vi "L0_Sum_Adder.vi"() -> ()   [LabVIEW 2009]
uses:
  Program Files/National Instruments/LabVIEW 2012/instr.lib/Agilent 8000 Series/Public/Configure/Configure Math (Binary Operation).vi
  <vilib>/Utility/file.llb/Write To Spreadsheet File (string).vi
  Program Files/National Instruments/LabVIEW 2012/instr.lib/Agilent 8000 Series/Public/Data/Low Level/Fetch Measurement (More).vi
  Program Files/National Instruments/LabVIEW 2012/instr.lib/Agilent 8000 Series/Agilent 8000 Series.lvlib
panel:
  in  "Channels Combinations":i32[](array[numeric])=[3, 12, 48, 96, 7, 28, 112, 15, 120, 31, 124, 63, 126, 127]
  out "error out":errorcluster={"status"=TRUE, "code"=-1073807343, "source"="VISA Open in Agilent 81150.lvlib:Initialize.vi->Set_Gen_Conf.vi->L0_Sum_Adder.vi"}
  in  "Voltage Array":dbl[](array[numeric])=[0.2, 0.4, 0.6, 0.8]
  in  "Osc":refnum<visa-resource-name>="Oscilloscope"
  in  "Generator":refnum<visa-resource-name>="generadorpulsos"
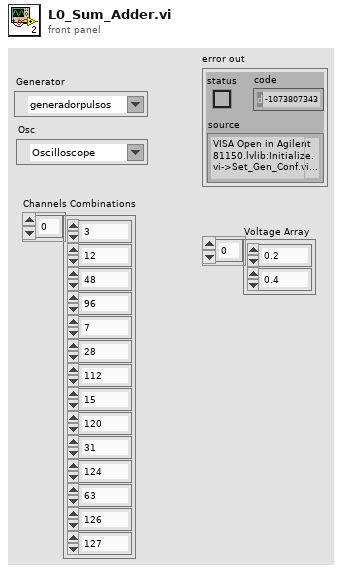
[diagram p1: front panel]
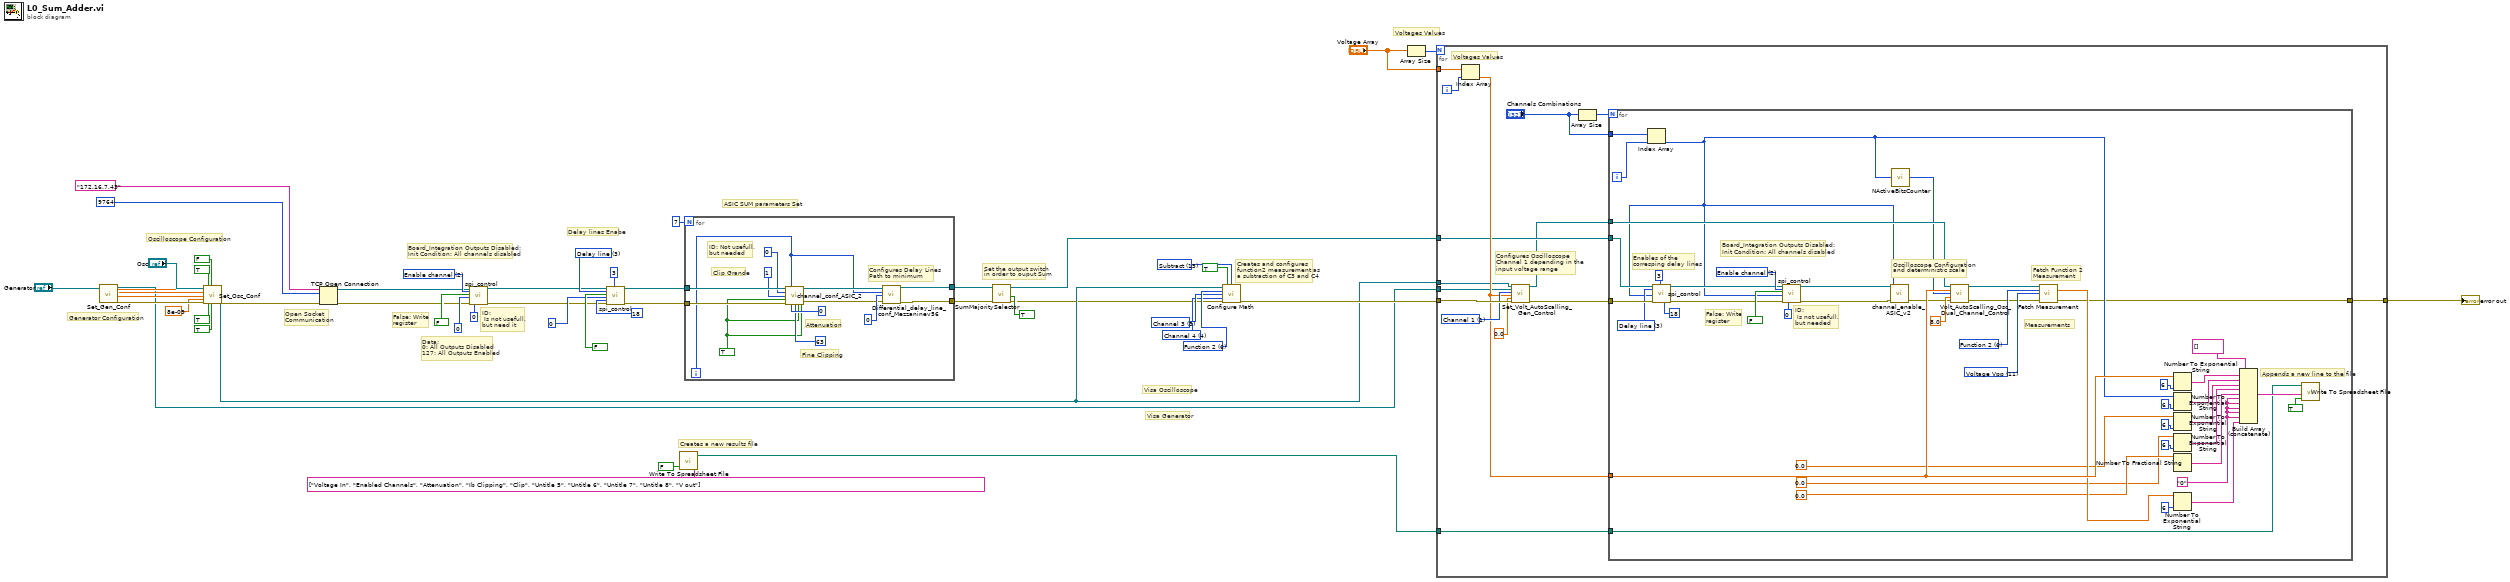
[diagram p0: block diagram]
diagram:
  w18 = u16 2 items=["Attenuation", "Clipping", "Enable channel", "Delay line", "ASIC"] ("Device")
  w21 = u16 3 items=["Attenuation", "Clipping", "Enable channel", "Delay line", "ASIC"] ("Device")
  w33 = u16 6 items=["Function 1"=5, "Function 2"=6, "Function 3"=7, "Function 4"=8] ("Math Channel (5: Function 1)")
  w34 = u16 15 items=["Add"=12, "Divide"=13, "Multiply"=14, "Subtract"=15, "Common Mode"=16, "Versus"=17] ("Math Operation (12: Add)")
  w32 = 3 items=["Channel 1"=1, "Channel 2"=2, "Channel 3"=3, "Channel 4"=4] ("Channel (1: Channel 1)")
  w31 = 4 items=["Channel 1"=1, "Channel 2"=2, "Channel 3"=3, "Channel 4"=4] ("Channel (1: Channel 1)")
  # "Creates and configures\nfunction2 measurement as\na subtraction of C3 and C4"
  # "Creates a new results file"
  # "Set the output switch\nin order to ouput Sum"
  # "ASIC SUM parameters Set"
  # "False: Write\nregister"
  # "Data:\n0: All Outputs Disabled\n127: All Outputs Enabled"
  # "ID:\n Is not usefull, \nbut need it"
  # "Board_Integration Outputs Disabled:\nInit Condition: All channels disabled"
  # "Delay lines Enabe"
  # "Open Socket\nCommunication"
  # "Visa Generator"
  # "Visa Oscilloscope"
  # "Oscilloscope Configuration"
  # "Voltages Values"
  # "Generator Configuration"
  n1 = call "Set_Gen_Conf.vi"("AWG VISA"="Generator") -> ("Amplitude 1 OUT"=w41:dbl, "VISA resource name out"=w26:refnum<visa-resource-name>, "Pulse Width in seconds 1 OUT"=w40:dbl, "Trigger Level 1"=w39:dbl, "error out"=w38:errorcluster)  [unwired: 11 in, 3 out]
  n2 = call "Set_Osc_Conf.vi"("VISA resource name"="Osc", "Amplitude IN"=w41, "Trigger Level IN"=w39, "Pulse Width in seconds IN"=w40, "Position 1"=8e-09, "error in (no error)"=w38, "Channel 1"=TRUE, "Channel 3"=TRUE, "Channel 2"=FALSE, "Channel 4"=TRUE) -> ("VISA resource name out"=w25:refnum<visa-resource-name>, "error out"=w15:errorcluster)  [unwired: 8 in]
  n3 = TCP Open Connection(address="172.16.7.43", remote port or service name=u16 9764, error in (no error)=w15) -> (connection ID=w14:refnum<k5>, error out=w13:errorcluster)  [unwired: 2 in]
  n4 = call "spi_control.vi"("connection ID"=w14, "Device"=w18, "Read/#write"=FALSE, "Data"=0, "error out 3"=w13, "Id in"=0) -> ("connection ID out"=w2:refnum<k5>, "error out 2"=w1:errorcluster)  [unwired: 6 in, 6 out]
  n5 = call "spi_control.vi"("connection ID"=w2, "Device"=w21, "Read/#write"=FALSE, "Data"=0, "Register or channel"=18, "error out 3"=w1, "chip delay"=3) -> ("connection ID out"=w11:refnum<k5>, "error out 2"=w12:errorcluster)  [unwired: 5 in, 6 out]
  n6 = call-poly <vilib>:"Write To Spreadsheet File.vi"("append to file? (new file:F)"=FALSE, "1D data"=string[] ["Voltage In", "Enabled Channels", "Attenuation", "Ib Clipping", "Clip", "Untitle 5", "Untitle 6", "Untitle 7", "Untitle 8", "V out"]) -> ("new file path (Not A Path if cancelled)"=w27:path)  [unwired: 6 in]
  n7 = for {
    N: 7 -> [_]
    tunnel: w12 -> [w62]
    tunnel: w11 -> [w61]
    tunnel: [w51] -> w7
    tunnel: [w52] -> w9
    i -> [w50]
    w56 = TRUE ("maj/sum")
    # "Configures Delay Lines\nPath to minimum"
    # "Attenuation"
    # "Fine Clipping"
    # "Clip Grande"
    # "ID: Not usefull,\nbut needed"
    n8 = call "channel_conf_ASIC_2.vi"("connection ID"=w61, "Ring"=w50, "Id in"=u32 0, "Clip_sel_b"=u32 1, "CompBuf_en_b"=w56, "error out"=w62, "Att gain"=u32 0, "Ib_ClipVb"=u32 63, "Clip_en_b"=w56, "Att_en_b"=w56) -> ("connection ID out"=w54:refnum<k5>, "error out 2"=w53:errorcluster)  [unwired: 1 in, 3 out]
    n9 = call "Differential_delay_line_conf_Mezzaninev56.vi"("connection ID"=w54, "channel"=w50, "Delay value"=u16 0, "error in (no error)"=w53) -> ("connection ID out"=w51:refnum<k5>, "error out 2"=w52:errorcluster)  [unwired: 4 in, 6 out]
  }
  n10 = call "SumMajoritySelector.vi"("On Sum\nOff Majority"=TRUE ("On Sum\nOff Majority"), "error in (no error)"=w9, "connection ID"=w7) -> ("error out"=w5:errorcluster, "connection ID out"=w6:refnum<k5>)  [unwired: 5 in]
  n11 = call-poly "Configure Math.vi"("VISA resource name"=w25, "Enable Math Channel (T:Enable)"=TRUE, "Math Operation (12: Add)"=w34, "Math Channel (5: Function 1)"=w33, "Math Operand (1: Channel 1)"=w32, "Math Operand (2: Channel 2)"=w31, "error in (no error)"=w5) -> ("error out"=w30:errorcluster)  [unwired: 7 in, 1 out]
  n12 = Array Size(array="Voltage Array") -> (size(s)=w37:i32)
  n13 = for {
    N: w37 -> [_]
    tunnel: w6 -> [w68]
    tunnel: w30 -> [w75]
    tunnel: "Voltage Array" -> [w77]
    tunnel: w27 -> [w72]
    tunnel: w26 -> [w70]
    tunnel: w25 -> [w69]
    tunnel: [w63] -> w3
    i -> [w76]
    w74 = 1 items=["Channel 1"=1, "Channel 2"=2, "Channel 3"=3, "Channel 4"=4] ("Channel")
    # "Configures Oscilloscope\nChannel 1 depending in the \ninput voltage range"
    # "Voltages Values"
    n14 = Index Array(array=w77, index=w76) -> (element=w73:dbl)
    n15 = call "Set_Volt_AutoScalling_Gen_Control.vi"("VISA Oscilloscope"=w69, "VISA Generator"=w70, "Channel"=w74, "Amplitude"=w73, "DC Offset"=0.0, "error in (no error)"=w75) -> ("VISA Oscilloscope"=w66:refnum<visa-resource-name>, "error out"=w67:errorcluster)  [unwired: 11 in, 1 out]
    n16 = Array Size(array="Channels Combinations") -> (size(s)=w65:i32)
    n17 = for {
      N: w65 -> [_]
      tunnel: w68 -> [w96]
      tunnel: w73 -> [w104]
      tunnel: w72 -> [w105]
      tunnel: w67 -> [w95]
      tunnel: w66 -> [w83]
      tunnel: "Channels Combinations" -> [w81]
      tunnel: [w78] -> w63
      i -> [w80]
      w89 = u16 2 items=["Attenuation", "Clipping", "Enable channel", "Delay line", "ASIC"] ("Device")
      w92 = u16 3 items=["Attenuation", "Clipping", "Enable channel", "Delay line", "ASIC"] ("Device")
      w111 = "0" ("F-format string")
      w121 = 11 items=["Rise Time", "Fall Time", "Frequency", "Period", "Voltage RMS(AC)", "Voltage RMS(DC)", "Voltage RMS (AC,cycle)", "Voltage RMS (DC,cycle)", "Voltage Max", "Voltage Min", "Voltage Middle", "Voltage Vpp", "Voltage High", "Voltage Low", "Voltage Average", "Voltage Average (cycle)", "Width Negative", "Width Positive", "Duty Cycle Positive", "Amplitude", "Overshoot", "Preshoot", "Voltage Base", "Voltage Upper", "Time Max", "Time Min", "Color Grade Crossing", "Color Grade Eye Width", "Color Grade Eye Height", "Color Grade Eye Q-Factory", "Color Grade Eye Duty Cycle Distortion(Percent)", "Color Grade Eye Duty Cycle Distortion(Time)", "Color Grade Eye Jitter(PP)", "Color Grade Eye Width(RMS)", "Cycle-cycle Duty Jitter(Rising)", "Cycle-cycle Duty Jitter(Falling)", "Cycle-cycle Jitter(Rising)", "Cycle-cycle Jitter(Falling)", "Cycle-cycle - Width", "Cycle-cycle + Width", "Date Rate", "Unit Interval", "FFT Delta Frequency", "FFT Delta Magnitude", "FFT Frequency", "FFT Magnitude", "Slew Rate", "Area (Entire Display)", "Area(Single Cycle)", "Duty Cycle (Rising)", "Duty Cycle (Falling)"] ("Measurement Function (0: Rise Time)")
      w122 = 6 items=["Channel 1"=1, "Channel 2"=2, "Channel 3"=3, "Channel 4"=4, "Function 1"=5, "Function 2"=6, "Function 3"=7, "Function 4"=8, "Memory 1"=9, "Memory 2"=10, "Memory 3"=11, "Memory 4"=12] ("Channel (1: Channel 1)")
      # "Appends a new line to the file"
      # "Fetch Function 2\nMeasurement"
      # "Enables of the\ncorresping delay lines"
      # "False: Write\nregister"
      # "ID:\n Is not usefull, \nbut needed"
      # "Board_Integration Outputs Disabled:\nInit Condition: All channels disabled"
      # "Measurements"
      # "Oscilloscope Configuration \nand deterministic scale"
      n18 = Index Array(array=w81, index=w80) -> (element=w79:i32)
      n19 = call "spi_control.vi"("connection ID"=w96, "Device"=w92, "Data"=w79, "Register or channel"=18, "error out 3"=w95, "chip delay"=3) -> ("connection ID out"=w87:refnum<k5>, "error out 2"=w86:errorcluster)  [unwired: 6 in, 6 out]
      n20 = call "spi_control.vi"("connection ID"=w87, "Device"=w89, "Read/#write"=FALSE, "Data"=w79, "error out 3"=w86, "Id in"=0) -> ("connection ID out"=w85:refnum<k5>, "error out 2"=w84:errorcluster)  [unwired: 6 in, 6 out]
      n21 = call "channel_enable_ASIC_v2.vi"("error in"=w84, "Channel Combination"=w79, "Connection ID in"=w85) -> ("error out"=w91:errorcluster)  [unwired: 7 in, 1 out]
      n22 = call "NActiveBitsCounter.vi"("Input Number"=w79) -> ("N High Bits"=w82:i32)
      n23 = call "Volt_AutoScalling_Osc_Dual_Channel_Control.vi"("VISA Oscilloscope"=w83, "Voltage In"=w104, "N Channels"=w82, "Offset Divider"=8.0, "error in"=w91) -> ("VISA resource name out"=w102:refnum<visa-resource-name>, "error out"=w100:errorcluster)  [unwired: 9 in]
      n24 = call-poly "Fetch Measurement.vi"("VISA resource name"=w102, "Channel (1: Channel 1)"=w122, "Measurement Function (0: Rise Time)"=w121, "error in (no error)"=w100) -> ("Measurement"=w101:dbl, "error out"=w78:errorcluster)  [unwired: 9 in, 1 out]
      n25 = Number To Exponential String(number=w104, precision (6)=i16 6) -> (E-format string=w112:string)  [unwired: 2 in]
      n26 = Number To Exponential String(number=w101, precision (6)=i16 6) -> (E-format string=w110:string)  [unwired: 2 in]
      n27 = Number To Exponential String(number=w79, precision (6)=i16 6) -> (E-format string=w120:string)  [unwired: 2 in]
      n28 = Number To Exponential String(number=0.0 ("Offset Divider"), precision (6)=i16 6) -> (E-format string=w119:string)  [unwired: 2 in]
      n29 = Number To Exponential String(number=0.0 ("Offset Divider"), precision (6)=i16 6) -> (E-format string=w117:string)  [unwired: 2 in]
      n30 = Number To Fractional String(number=0.0 ("Offset Divider")) -> (F-format string=w113:string)  [unwired: 3 in]
      n31 = Build Array (concatenate)(string[] [] ("array"), w112, w120, w119, w117, w113, w111, w111, w111, w111, w111, w110) -> (w106:string[])
      n32 = call-poly <vilib>:"Write To Spreadsheet File.vi"("append to file? (new file:F)"=TRUE, "1D data"=w106, "file path (dialog if empty)"=w105) -> ()  [unwired: 5 in, 1 out]
    }
  }
  "error out" <- w3
